vi "byte2data.vi"(1 "string":string, 2 "Read":bool) -> (3 "OK":bool, 5 "vacuo (mBar)":dbl, 6 "RTD-chamber (ºC)":sgl format="%0.2f", 7 "P01 (Bar)":dbl, 8 "P02 (Bar)":dbl, 9 "RTD-01 (ºC)":sgl format="%0.2f", 10 "RTD-02 (ºC)":sgl format="%0.2f")   [LabVIEW 2011]
uses:
  <vilib>/Utility/TradDaqScaling.llb/Convert RTD Reading (scaler).vi
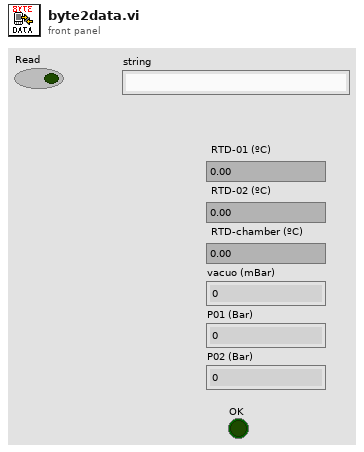
[diagram p1: front panel]
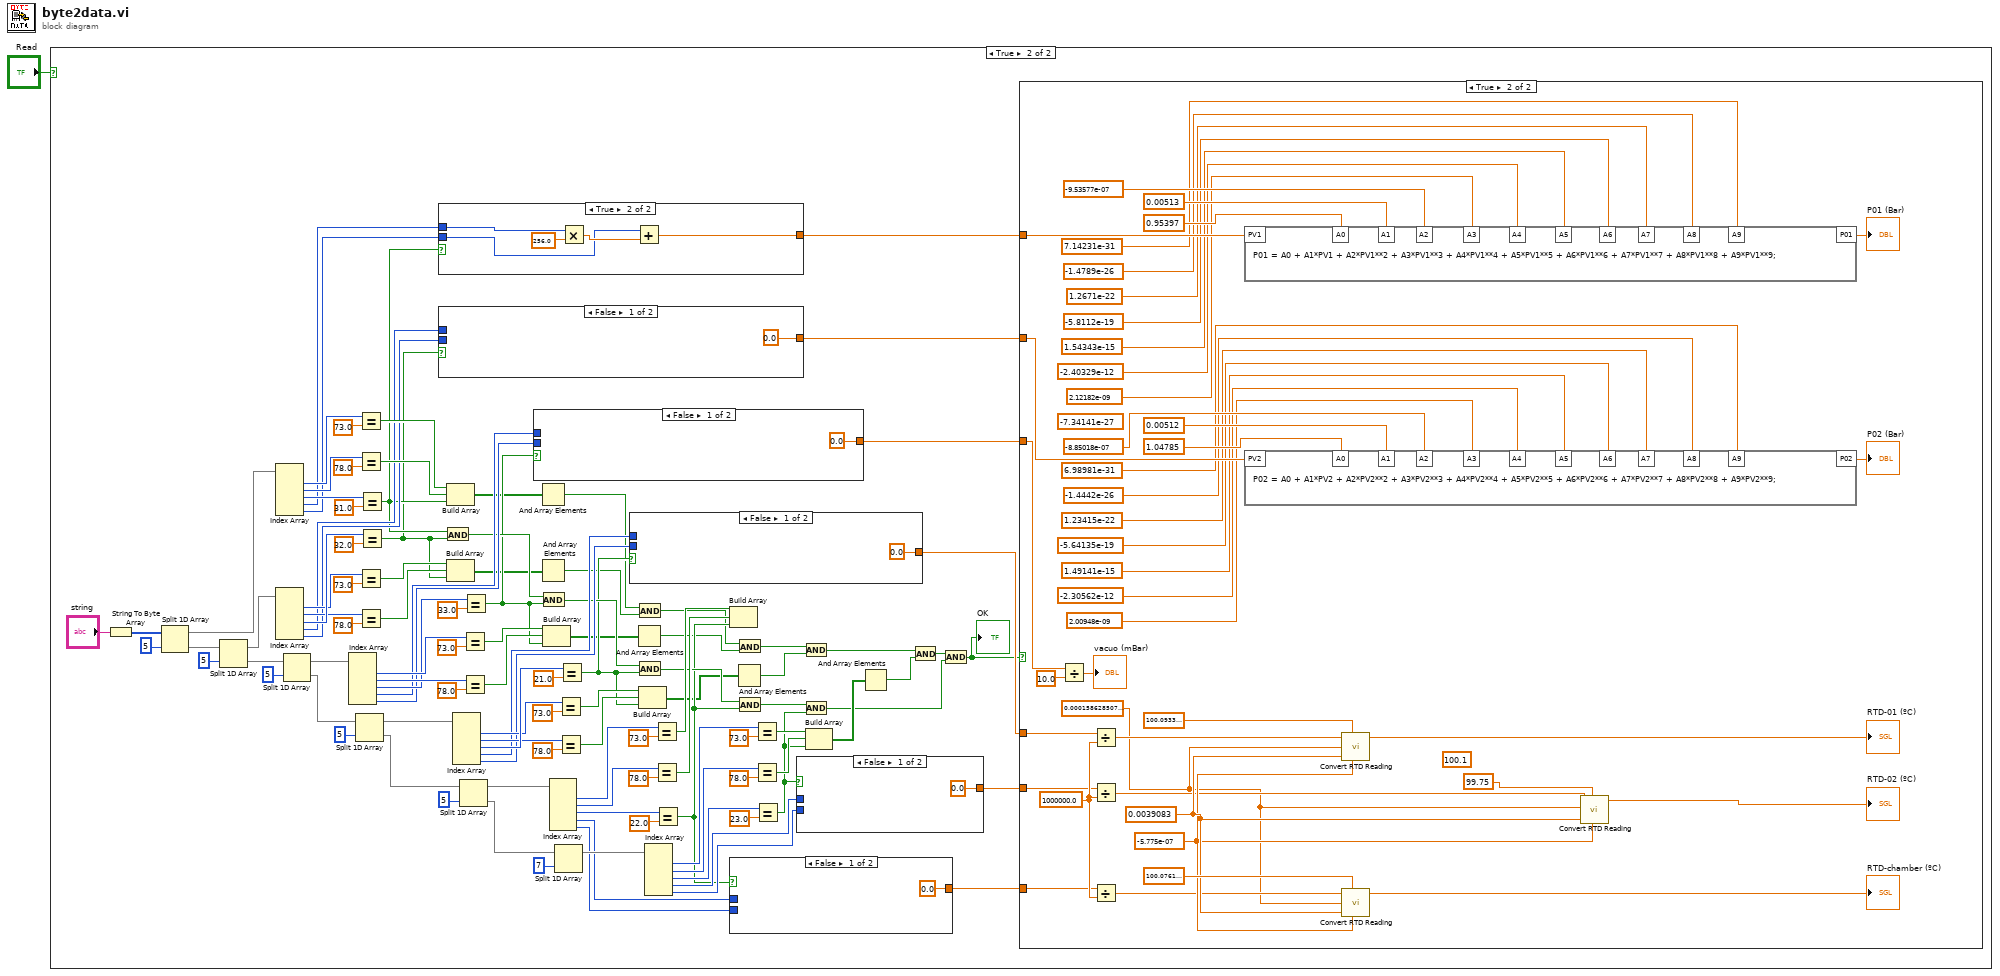
[diagram p0: block diagram]
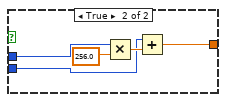
[diagram p4: hidden frame]
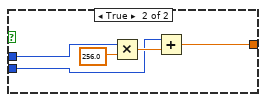
[diagram p5: hidden frame]
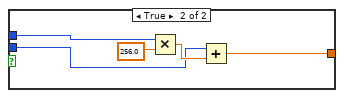
[diagram p6: hidden frame]
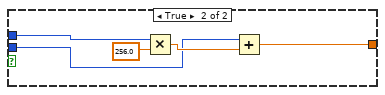
[diagram p7: hidden frame]
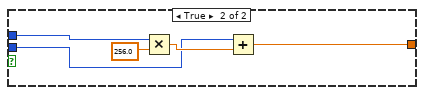
[diagram p8: hidden frame]
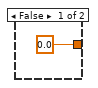
[diagram p9: hidden frame]
diagram:
  n1 = case shown="True" "Read" {
    frame False {
    }
    frame True {
      n2 = String To Byte Array(string="string") -> (unsigned byte array=w101:u8[])
      n3 = Split 1D Array(array=w101, index=5 ("Numeric 2")) -> (first subarray=w94:u8[], second subarray=w102:u8[])
      n4 = Split 1D Array(array=w102, index=5 ("Numeric 2")) -> (first subarray=w83:u8[], second subarray=w103:u8[])
      n5 = Index Array(array=w94) -> (element #1=w99:u8, element #2=w98:u8, element #3=w97:u8, element #4=w46:u8, element #5=w45:u8)  [unwired: 5 in]
      n6 = Index Array(array=w83) -> (element #1=w85:u8, element #2=w86:u8, element #3=w87:u8, element #4=w44:u8, element #5=w43:u8)  [unwired: 5 in]
      n7 = Split 1D Array(array=w103, index=5 ("Numeric 2")) -> (first subarray=w74:u8[], second subarray=w105:u8[])
      n8 = Index Array(array=w74) -> (element #1=w81:u8, element #2=w80:u8, element #3=w79:u8, element #4=w42:u8, element #5=w41:u8)  [unwired: 5 in]
      n9 = Split 1D Array(array=w105, index=5 ("Numeric 2")) -> (first subarray=w65:u8[], second subarray=w106:u8[])
      n10 = Equal?(x=w99, y=73.0) -> (x = y?=w93:bool)
      n11 = Equal?(x=w98, y=78.0) -> (x = y?=w92:bool)
      n12 = Equal?(x=w85, y=73.0) -> (x = y?=w90:bool)
      n13 = Equal?(x=w86, y=78.0) -> (x = y?=w91:bool)
      n14 = Equal?(x=w97, y=31.0) -> (x = y?=w23:bool)
      n15 = Equal?(x=w87, y=32.0) -> (x = y?=w22:bool)
      n16 = case shown="True" w23 {
        tunnel: w46 -> [_ w189]
        tunnel: w45 -> [_ w188]
        tunnel: [0.0 w187] -> w33
        frame False {
        }
        frame True {
          n17 = Multiply(x=w189, y=256.0) -> (x*y=w190:dbl)
          n18 = Add(x=w188, y=w190) -> (x+y=w187:dbl)
        }
      }
      n19 = case shown="False" w22 {
        tunnel: w44 -> [_ w183]
        tunnel: w43 -> [_ w182]
        tunnel: [0.0 w181] -> w32
        frame False {
        }
        frame True {
          n20 = Multiply(x=w183, y=256.0) -> (x*y=w184:dbl)
          n21 = Add(x=w182, y=w184) -> (x+y=w181:dbl)
        }
      }
      n22 = And(x=w23, y=w22) -> (x .and. y?=w27:bool)
      n23 = Build Array(w93, w92, w23) -> (w17:bool[])
      n24 = Build Array(w90, w91, w22) -> (w16:bool[])
      n25 = Index Array(array=w65) -> (element #1=w67:u8, element #2=w68:u8, element #3=w69:u8, element #4=w40:u8, element #5=w39:u8)  [unwired: 5 in]
      n26 = Split 1D Array(array=w106, index=5 ("Numeric 2")) -> (first subarray=w56:u8[], second subarray=w112:u8[])
      n27 = Equal?(x=w81, y=73.0) -> (x = y?=w76:bool)
      n28 = Equal?(x=w80, y=78.0) -> (x = y?=w75:bool)
      n29 = Equal?(x=w79, y=33.0) -> (x = y?=w21:bool)
      n30 = case shown="False" w21 {
        tunnel: w42 -> [_ w177]
        tunnel: w41 -> [_ w176]
        tunnel: [0.0 w175] -> w31
        frame False {
        }
        frame True {
          n31 = Multiply(x=w177, y=256.0) -> (x*y=w178:dbl)
          n32 = Add(x=w176, y=w178) -> (x+y=w175:dbl)
        }
      }
      n33 = And Array Elements(Boolean array=w17) -> (logical AND=w8:bool)
      n34 = And Array Elements(Boolean array=w16) -> (logical AND=w9:bool)
      n35 = And(x=w27, y=w21) -> (x .and. y?=w26:bool)
      n36 = Build Array(w76, w75, w21) -> (w15:bool[])
      n37 = Index Array(array=w56) -> (element #1=w63:u8, element #2=w62:u8, element #3=w61:u8, element #4=w38:u8, element #5=w37:u8)  [unwired: 5 in]
      n38 = Split 1D Array(array=w112, index=7 ("Numeric 2")) -> (first subarray=w47:u8[])  [unwired: 1 out]
      n39 = Equal?(x=w67, y=73.0) -> (x = y?=w72:bool)
      n40 = Equal?(x=w68, y=78.0) -> (x = y?=w73:bool)
      n41 = Equal?(x=w69, y=21.0) -> (x = y?=w20:bool)
      n42 = case shown="False" w20 {
        tunnel: w40 -> [_ w171]
        tunnel: w39 -> [_ w170]
        tunnel: [0.0 w169] -> w30
        frame False {
        }
        frame True {
          n43 = Multiply(x=w171, y=256.0) -> (x*y=w172:dbl)
          n44 = Add(x=w170, y=w172) -> (x+y=w169:dbl)
        }
      }
      n45 = And Array Elements(Boolean array=w15) -> (logical AND=w10:bool)
      n46 = And(x=w8, y=w9) -> (x .and. y?=w7:bool)
      n47 = And(x=w26, y=w20) -> (x .and. y?=w25:bool)
      n48 = Build Array(w72, w73, w20) -> (w14:bool[])
      n49 = Index Array(array=w47) -> (element #1=w49:u8, element #2=w50:u8, element #3=w51:u8, element #4=w36:u8, element #5=w35:u8)  [unwired: 5 in]
      n50 = Equal?(x=w63, y=73.0) -> (x = y?=w58:bool)
      n51 = Equal?(x=w62, y=78.0) -> (x = y?=w57:bool)
      n52 = Equal?(x=w61, y=22.0) -> (x = y?=w19:bool)
      n53 = Build Array(w58, w57, w19) -> ()  [unwired: 1 out]
      n54 = case shown="False" w19 {
        tunnel: w38 -> [_ w165]
        tunnel: w37 -> [_ w164]
        tunnel: [0.0 w163] -> w29
        frame False {
        }
        frame True {
          n55 = Multiply(x=w165, y=256.0) -> (x*y=w166:dbl)
          n56 = Add(x=w164, y=w166) -> (x+y=w163:dbl)
        }
      }
      n57 = And Array Elements(Boolean array=w14) -> (logical AND=w11:bool)
      n58 = And(x=w7, y=w10) -> (x .and. y?=w6:bool)
      n59 = And(x=w25, y=w19) -> (x .and. y?=w24:bool)
      n60 = Equal?(x=w49, y=73.0) -> (x = y?=w54:bool)
      n61 = Equal?(x=w50, y=78.0) -> (x = y?=w55:bool)
      n62 = Equal?(x=w51, y=23.0) -> (x = y?=w18:bool)
      n63 = case shown="False" w18 {
        tunnel: w36 -> [_ w159]
        tunnel: w35 -> [_ w158]
        tunnel: [0.0 w157] -> w28
        frame False {
        }
        frame True {
          n64 = Multiply(x=w159, y=256.0) -> (x*y=w160:dbl)
          n65 = Add(x=w158, y=w160) -> (x+y=w157:dbl)
        }
      }
      n66 = And(x=w6, y=w11) -> (x .and. y?=w5:bool)
      n67 = And(x=w24, y=w18) -> (x .and. y?=w3:bool)
      n68 = Build Array(w54, w55, w18) -> (w13:bool[])
      n69 = And Array Elements(Boolean array=w13) -> (logical AND=w12:bool)
      n70 = And(x=w5, y=w12) -> (x .and. y?=w4:bool)
      n71 = And(x=w4, y=w3) -> (x .and. y?=w2:bool)
      "OK" <- w2
      n72 = case shown="True" w2 {
        tunnel: w33 -> [_ w136]
        tunnel: w32 -> [_ w125]
        tunnel: w31 -> [_ w140]
        tunnel: w30 -> [_ w139]
        tunnel: w29 -> [_ w138]
        tunnel: w28 -> [_ w137]
        frame False {
        }
        frame True {
          (unwired) 100.1 ("Ro 3")
          (unwired) -7.34141e-27 ("input variable")
          w152 = 1000000.0 ("y")
          w143 = sgl 0.0001586285 ("Iex")
          w150 = -5.775e-07
          w151 = 0.0039083
          n73 = Divide(x=w140, y=10.0) -> (x/y=→"vacuo (mBar)":dbl)
          n74 = Divide(x=w139, y=w152) -> (x/y=w146:dbl)
          n75 = Divide(x=w137, y=w152) -> (x/y=w144:dbl)
          n76 = Divide(x=w138, y=w152) -> (x/y=w145:dbl)
          n77 = formula code="P01 = A0 + A1*PV1 + A2*PV1**2 + A3*PV1**3 + A4*PV1**4 + A5*PV1**5 + A6*PV1**6 + A7*PV1**7 + A8*PV1**8 + A9*PV1**9;"("PV1"=w136, "A0"=0.95397 ("input variable"), "A1"=0.00513 ("input variable"), "A2"=-9.53577e-07 ("input variable"), "A3"=2.12182e-09 ("input variable"), "A4"=-2.40329e-12 ("input variable"), "A5"=1.54343e-15 ("input variable"), "A6"=-5.8112e-19 ("input variable"), "A7"=1.2671e-22 ("input variable"), "A8"=-1.4789e-26 ("input variable"), "A9"=7.14231e-31 ("input variable")) -> ("P01"=→"P01 (Bar)":dbl)
          n78 = formula code="P02 = A0 + A1*PV2 + A2*PV2**2 + A3*PV2**3 + A4*PV2**4 + A5*PV2**5 + A6*PV2**6 + A7*PV2**7 + A8*PV2**8 + A9*PV2**9;"("PV2"=w125, "A0"=1.04785 ("input variable"), "A1"=0.00512 ("input variable"), "A2"=-8.85018e-07 ("input variable"), "A3"=2.00948e-09 ("input variable"), "A4"=-2.30562e-12 ("input variable"), "A5"=1.49141e-15 ("input variable"), "A6"=-5.64135e-19 ("input variable"), "A7"=1.23415e-22 ("input variable"), "A8"=-1.4442e-26 ("input variable"), "A9"=6.98981e-31 ("input variable")) -> ("P02"=→"P02 (Bar)":dbl)
          n79 = call-poly <vilib>:"Convert RTD Reading.vi"("RTDvolts"=w146, "Ro"=sgl 100.0934, "Iex"=w143, "A"=w151, "B"=w150) -> ("RTDtemp"=→"RTD-01 (ºC)":sgl)  [unwired: 2 in]
          n80 = call-poly <vilib>:"Convert RTD Reading.vi"("RTDvolts"=w145, "Ro"=sgl 100.0761 ("Ro 2"), "Iex"=w143, "A"=w151, "B"=w150) -> ("RTDtemp"=→"RTD-chamber (ºC)":sgl)  [unwired: 2 in]
          n81 = call-poly <vilib>:"Convert RTD Reading.vi"("RTDvolts"=w144, "Ro"=99.75 ("Ro 3"), "Iex"=w143, "A"=w151, "B"=w150) -> ("RTDtemp"=→"RTD-02 (ºC)":sgl)  [unwired: 2 in]
        }
      }
    }
  }
